vi "CreateChannels_TC.vi"(8 "error in":errorcluster) -> (0 "error out":errorcluster, 3 "task out":refnum<k21>)   [LabVIEW 2017]
uses:
  <vilib>/DAQmx/create/channels.llb/DAQmx Create Channel (AI-Temperature-Thermocouple).vi
  <resource>/objmgr/daqmx.rc
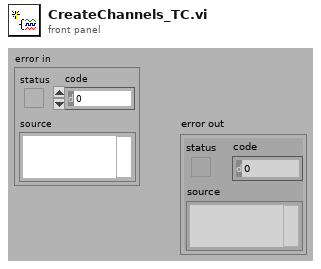
[diagram p1: front panel]
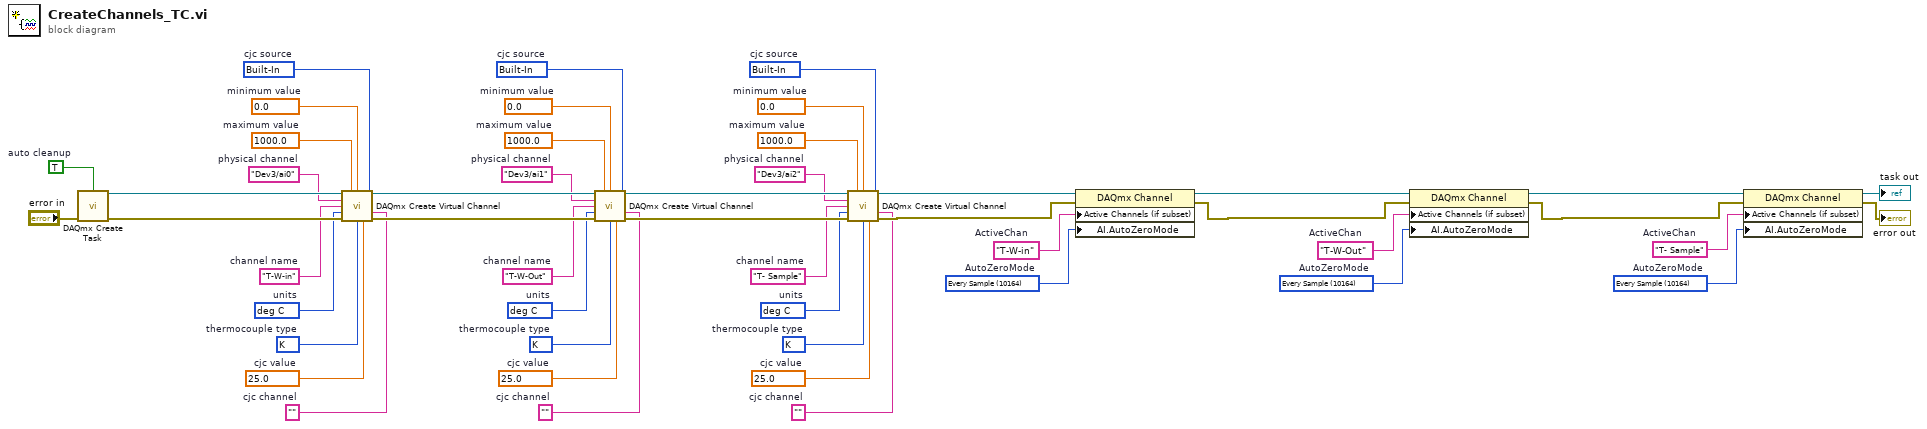
[diagram p0: block diagram]
diagram:
  w1 = 10164 items=["None"=10230, "Once"=10244, "Every Sample"=10164]  # AutoZeroMode
  w5 = "T- Sample"  # ActiveChan
  w6 = 10164 items=["None"=10230, "Once"=10244, "Every Sample"=10164]  # AutoZeroMode
  w9 = "T-W-Out"  # ActiveChan
  w10 = 10164 items=["None"=10230, "Once"=10244, "Every Sample"=10164]  # AutoZeroMode
  w13 = "T-W-in"  # ActiveChan
  w14 = 10200 items=["Built-In"=10200, "Constant Value"=10116, "Channel"=10113]  # cjc source
  w16 = ""  # cjc channel
  w17 = 25.0  # cjc value
  w18 = 10073 items=["J"=10072, "K"=10073, "N"=10077, "R"=10082, "S"=10085, "T"=10086, "B"=10047, "E"=10055]  # thermocouple type
  w19 = 10143 items=["deg C"=10143, "deg F"=10144, "Kelvins"=10325, "deg R"=10145, "From Custom Scale"=10065]  # units
  w15 = "T- Sample"  # channel name
  w21 = 0.0  # minimum value
  w22 = 1000.0  # maximum value
  w23 = "Dev3/ai2"  # physical channel
  w25 = 10200 items=["Built-In"=10200, "Constant Value"=10116, "Channel"=10113]  # cjc source
  w27 = ""  # cjc channel
  w28 = 25.0  # cjc value
  w29 = 10073 items=["J"=10072, "K"=10073, "N"=10077, "R"=10082, "S"=10085, "T"=10086, "B"=10047, "E"=10055]  # thermocouple type
  w30 = 10143 items=["deg C"=10143, "deg F"=10144, "Kelvins"=10325, "deg R"=10145, "From Custom Scale"=10065]  # units
  w26 = "T-W-Out"  # channel name
  w32 = 0.0  # minimum value
  w33 = 1000.0  # maximum value
  w34 = "Dev3/ai1"  # physical channel
  w36 = 10200 items=["Built-In"=10200, "Constant Value"=10116, "Channel"=10113]  # cjc source
  w38 = ""  # cjc channel
  w39 = 25.0  # cjc value
  w40 = 10073 items=["J"=10072, "K"=10073, "N"=10077, "R"=10082, "S"=10085, "T"=10086, "B"=10047, "E"=10055]  # thermocouple type
  w41 = 10143 items=["deg C"=10143, "deg F"=10144, "Kelvins"=10325, "deg R"=10145, "From Custom Scale"=10065]  # units
  w37 = "T-W-in"  # channel name
  w43 = 0.0  # minimum value
  w44 = 1000.0  # maximum value
  w45 = "Dev3/ai0"  # physical channel
  w47 = TRUE  # auto cleanup
  n1 = call <vilib>:"DAQmx Create Task.vi"("auto cleanup"=w47, "error in"="error in") -> ("task out"=w46:refnum<k21>, "error out"=w48:errorcluster)  [unwired: 12 in]
  n2 = call-poly <vilib>:"DAQmx Create Virtual Channel.vi"("task in"=w46, "maximum value"=w44, "minimum value"=w43, "physical channels"=w45, "cjc source"=w36, "name to assign"=w37, "units"=w41, "cjc channel"=w38, "error in"=w48, "thermocouple type"=w40, "cjc value"=w39) -> ("task out"=w35:refnum<k21>, "error out"=w42:errorcluster)  [unwired: 3 in]
  n3 = call-poly <vilib>:"DAQmx Create Virtual Channel.vi"("task in"=w35, "maximum value"=w33, "minimum value"=w32, "physical channels"=w34, "cjc source"=w25, "name to assign"=w26, "units"=w30, "cjc channel"=w27, "error in"=w42, "thermocouple type"=w29, "cjc value"=w28) -> ("task out"=w24:refnum<k21>, "error out"=w31:errorcluster)  [unwired: 3 in]
  n4 = call-poly <vilib>:"DAQmx Create Virtual Channel.vi"("task in"=w24, "maximum value"=w22, "minimum value"=w21, "physical channels"=w23, "cjc source"=w14, "name to assign"=w15, "units"=w19, "cjc channel"=w16, "error in"=w31, "thermocouple type"=w18, "cjc value"=w17) -> ("task out"=w11:refnum<k21>, "error out"=w20:errorcluster)  [unwired: 3 in]
  n5 = property class="DAQmx Channel"(reference=w11, error in=w20, "Active Channels (if subset)"=w13, "AI.AutoZeroMode"=w10) -> (reference out=w7:refnum<k21>, error out=w12:errorcluster)
  n6 = property class="DAQmx Channel"(reference=w7, error in=w12, "Active Channels (if subset)"=w9, "AI.AutoZeroMode"=w6) -> (reference out=w2:refnum<k21>, error out=w8:errorcluster)
  n7 = property class="DAQmx Channel"(reference=w2, error in=w8, "Active Channels (if subset)"=w5, "AI.AutoZeroMode"=w1) -> (reference out=→"task out":refnum<k21>, error out=→"error out":errorcluster)
